vi "Get Cursor Position Reverse.vi"(8 "Logarithm?":bool, 9 "Inverted?":bool, 10 "Range":cluster{"Max":sgl, "Min":sgl}, 11 "Cursor Value In":sgl) -> (3 "Cursor Value Out":sgl)   [LabVIEW 2017, in "3D Plot.lvclass"]
uses:
  <vilib>/Math Plots/3D Math Plots/3D Plot/3D Plot/3D Plot.lvclass
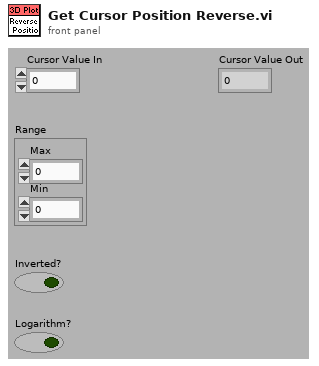
[diagram p1: front panel]
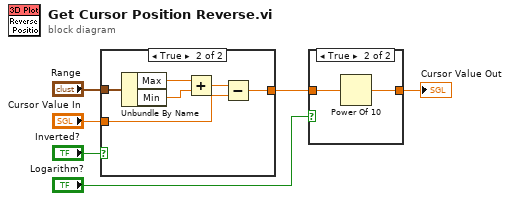
[diagram p0: block diagram]
diagram:
  n1 = case shown="True" "Inverted?" {
    tunnel: "Cursor Value In" -> [w7 w9]
    tunnel: [w7 w8] -> w5
    tunnel: "Range" -> [_ w13]
    frame False {
    }
    frame True {
      n2 = Unbundle By Name(w13) -> ("Max"=w12:sgl, "Min"=w11:sgl)
      n3 = Add(x=w12, y=w11) -> (x+y=w10:sgl)
      n4 = Subtract(x=w10, y=w9) -> (x-y=w8:sgl)
    }
  }
  n5 = case shown="True" "Logarithm?" {
    tunnel: w5 -> [w14 w16]
    tunnel: [w14 w15] -> w6
    frame False {
    }
    frame True {
      n6 = Power Of 10(x=w16) -> (10^x=w15:sgl)
    }
  }
  "Cursor Value Out" <- w6
